vi "DigiComm_TX.vi"(6 "filter parameters":T1={"Alpha"=0.5, "Filter Length"=6, "TX Filter"=enum."Root Raised Cos"} {"Alpha" format="%.2f"}, 7 "Num of Symbols":i32=100, 8 "Mapping Parameters":T2={"Modulation Order (M)"=2, "Modulation Type"=0, "Samples per Symbol"=8} {"Modulation Type" items=["PSK", "QAM"]}) -> (2 "input bit stream":i16[](array[numeric]), 3 "input complex waveform":T3 caption="output complex waveform" {"Y" format="%.3f"; "dt" format="%^.2e"; "t0" format="%.4f"})   [LabVIEW 2011]
uses:
  <vilib>/addons/Modulation/Analog/controls/Complex Data Waveform.ctl
  subVIs_Dcomm_offered/FilterCoefficient.ctl
  <vilib>/addons/Modulation/niDMT.lvlib
  <vilib>/addons/Modulation/niAMT.lvlib
panel:
  out "TX pulse shaping filter":dbl[](graph)
  out "Constellation Graph":T4(graph) caption="Tx Signal Constellation"
  # "Lab 2(b): Digital Communication (TX)"
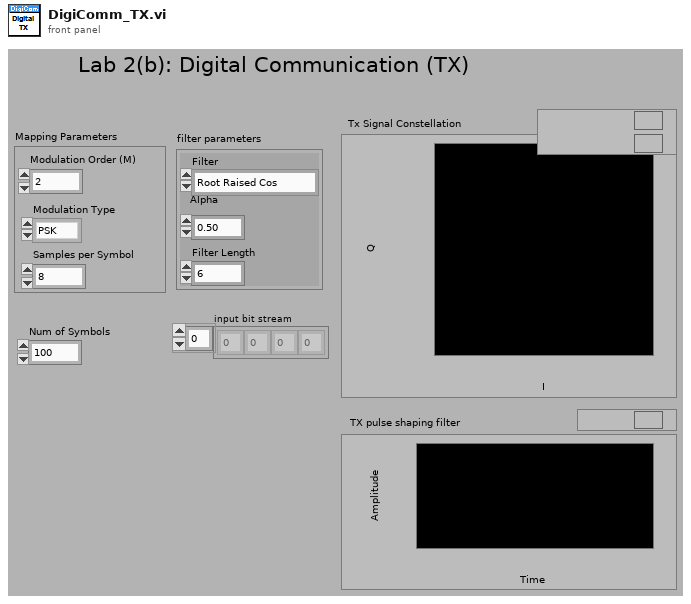
[diagram p1: front panel]
types:
  T1 = typedef "FilterCoefficient.ctl" = cluster{"Alpha":dbl, "Filter Length":i32, "TX Filter":enum16{"Root Raised Cos", "Raised Cos", "Rectangular"}}
  T2 = cluster{"Modulation Order (M)":i32, "Modulation Type":u16, "Samples per Symbol":i32}
  T3 = typedef "niAMT.lvlib/Complex Data Waveform.ctl" = cluster{"t0":dbl, "dt":dbl, "Y":cdb[]}
  T4 = cluster{"constellation":dbl[], "oversampled data":dbl[]}[]
  T5 = cluster{"samples per symbol (16)":i32, "symbol map":cdb[]}
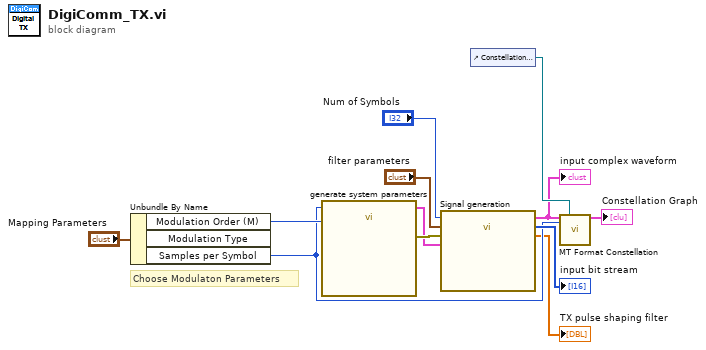
[diagram p0: block diagram]
diagram:
  # "Choose Modulaton Parameters"
  n1 = Unbundle By Name("Mapping Parameters") -> ("Modulation Order (M)"=w4:i32, "Samples per Symbol"=w3:i32)  [unwired: 1 out]
  n2 = call "generate system parameters.vi"("M-PSK"=w4, "samples per symbol"=w3) -> ("error out"=w10:errorcluster, "system parameters"=w8:T5)  [unwired: 8 in]
  n3 = call "Signal generation.vi"("system parameters"=w8, "error in (no error)"=w10, "filter parameters"="filter parameters", "NumOfSymbols"="Num of Symbols") -> ("pulse shaping filter coefficients"=→"TX pulse shaping filter":dbl[], "input bit stream"=→"input bit stream":i16[], "output complex waveform"=w9:T3)  [unwired: 4 in, 1 out]
  "input complex waveform" <- w9
  n4 = control-ref of="Constellation Graph"() -> (w12:refnum<vi>)
  n5 = call <vilib>:"MT Format Constellation.vi"("waveform"=w9, "constellation reference"=w12, "samples per symbol"=w3) -> ("constellation graph"=→"Constellation Graph":T4)  [unwired: 11 in, 1 out]
